vi "UtilityLib.TCPBufferSize.vi"(8 "error in (no error)":errorcluster, 10 "buffer size (8192)":i32=8192, 11 "connection in":refnum<k5>) -> (0 "error out":errorcluster, 3 "connection out":refnum<k5>)   [LabVIEW 2014, in "UtilityLib.lvlib"]
doc: "Sets the buffer size for TCP connections."
uses:
  UtilityLib.lvlib
  wsock32.dll
panel:
  out "setsockopt result":i32
  # "Turn TCP_NODELAY on or off on the given network refnum."
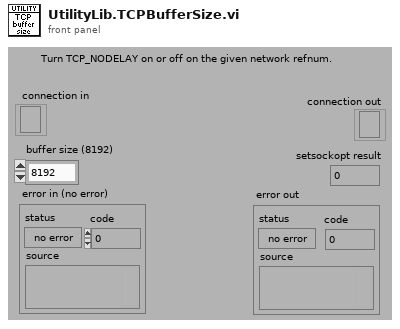
[diagram p1: front panel]
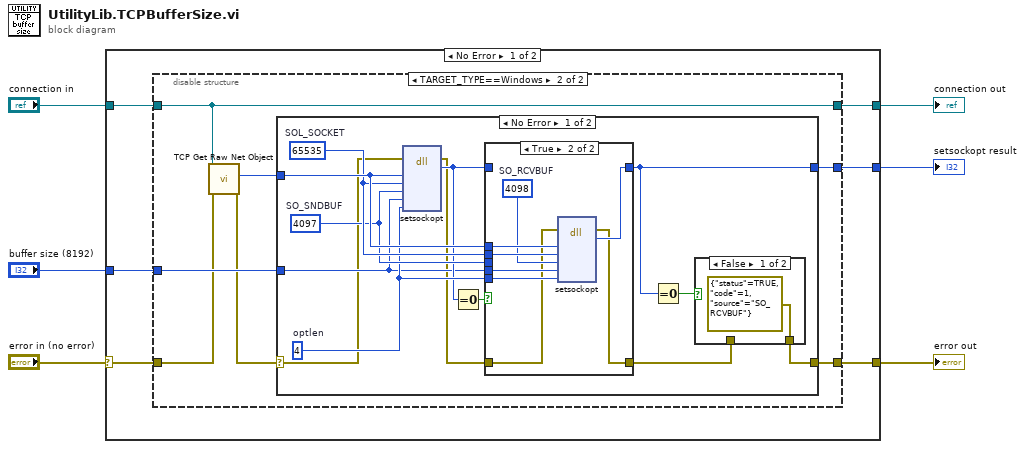
[diagram p0: block diagram]
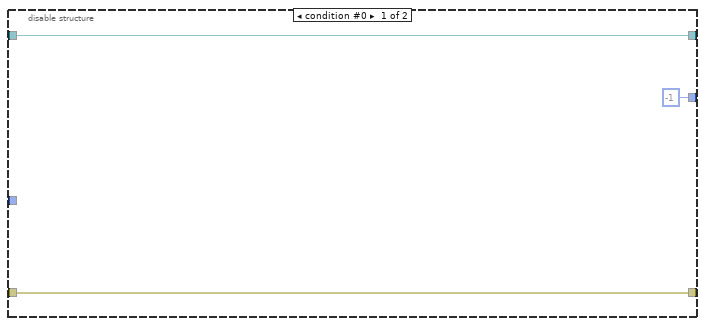
[diagram p2: hidden frame]
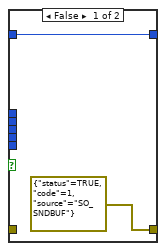
[diagram p4: hidden frame]
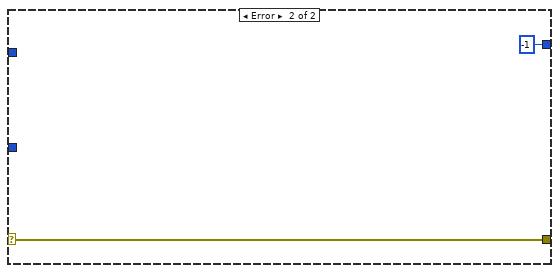
[diagram p5: hidden frame]
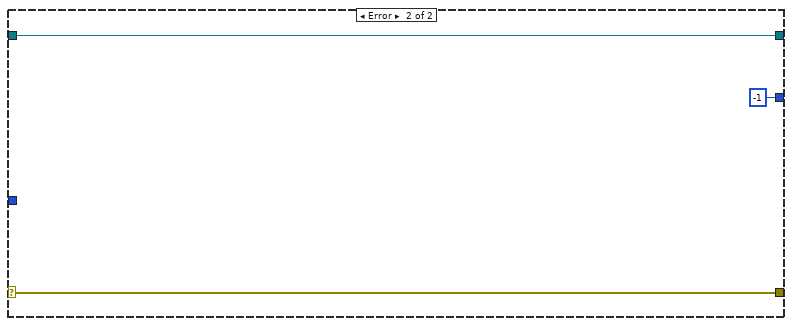
[diagram p6: hidden frame]
diagram:
  n1 = case shown="No Error" "error in (no error)" {
    selector: "error in (no error)" -> [w10 w52]
    tunnel: "connection in" -> [w12 w51]
    tunnel: [w9 w52] -> w4
    tunnel: [w11 w51] -> w3
    tunnel: "buffer size (8192)" -> [w8 _]
    tunnel: [w7 -1 ("return value")] -> w1
    frame No Error {
      n2 = disable-structure shown="TARGET_TYPE==Windows" {
        disable-tunnel: w12 -> [w15 w21]
        disable-tunnel: [w15 w21] -> w11
        disable-tunnel: w10 -> [w14 w18]
        disable-tunnel: [w14 w20] -> w9
        disable-tunnel: w8 -> [_ w19]
        disable-tunnel: [-1 ("return value") w16] -> w7
        frame condition #0 {
        }
        frame condition #1 (active) {
          n3 = call <vilib>:"TCP Get Raw Net Object.vi"("error in (no error)"=w18, "connection ID"=w21) -> ("error out"=w17:errorcluster, "raw net object"=w22:u64)  [unwired: 7 in, 1 out]
          n4 = case shown="No Error" w17 {
            selector: w17 -> [w24 w48]
            tunnel: [w29 w48] -> w20
            tunnel: w22 -> [w34 _]
            tunnel: [w27 -1] -> w16
            tunnel: w19 -> [w25 _]
            frame No Error {
              w32 = 4097  # SO_SNDBUF
              w33 = 65535  # SOL_SOCKET
              w31 = 4  # optlen
              n5 = dll-call lib="wsock32.dll" fn="setsockopt"(error in=w24, "s"=w34, "level"=w33, "optname"=w32, "optval"=w25, "optlen"=w31) -> (error out=w23:errorcluster, "return value"=w30:i32)  [unwired: 7 in, 1 out]
              n6 = Equal To 0?(x=w30) -> (x = 0?=w35:bool)
              n7 = case shown="True" w35 {
                tunnel: w23 -> [_ w41]
                tunnel: [errorcluster {"status"=TRUE, "code"=1, "source"="SO_SNDBUF"} ("error in (no error)") w40] -> w28
                tunnel: w34 -> [_ w47]
                tunnel: w33 -> [_ w46]
                tunnel: w32 -> [_ _]
                tunnel: w25 -> [_ w45]
                tunnel: w31 -> [_ w44]
                tunnel: [w39 w42] -> w27
                tunnel: w30 -> [w39 _]
                frame False {
                }
                frame True {
                  w43 = 4098  # SO_RCVBUF
                  n8 = dll-call lib="wsock32.dll" fn="setsockopt"(error in=w41, "s"=w47, "level"=w46, "optname"=w43, "optval"=w45, "optlen"=w44) -> (error out=w40:errorcluster, "return value"=w42:i32)  [unwired: 7 in, 1 out]
                }
              }
              n9 = Equal To 0?(x=w27) -> (x = 0?=w26:bool)
              n10 = case shown="False" w26 {
                tunnel: [errorcluster {"status"=TRUE, "code"=1, "source"="SO_RCVBUF"} ("error in (no error)") w37] -> w29
                tunnel: w28 -> [_ w37]
                frame False {
                }
                frame True {
                }
              }
            }
            frame Error {
            }
          }
        }
      }
    }
    frame Error {
    }
  }
  "connection out" <- w3
  "error out" <- w4
  "setsockopt result" <- w1
